vi "Send SYNC Pulse.vi"(8 "error in":errorcluster, 10 "Master?":bool=TRUE, 11 "FPGA Session":T1) -> (0 "error out":errorcluster, 3 "FPGA Session":T1)   [LabVIEW 2011, in "FlexRIO Host Library (User).lvlib"]
uses:
  FlexRIO Host Library (User).lvlib
  Session/FPGA Session Ref.ctl
  <vilib>/rvi/interface/nirviReadWriteControl/nirviReadWriteControl.xnode
  Zeiss Acquisition Demo/FPGA Bitfiles/FlexRIODigitizer_FPGABoard_Acquire_Rev2.lvbitx
  <vilib>/rvi/errors/niLvFpgaMergeErrorWithErrorCode.vi
  <vilib>/rvi/errors/niLvFpgaAdjustHostInterfaceError.vi
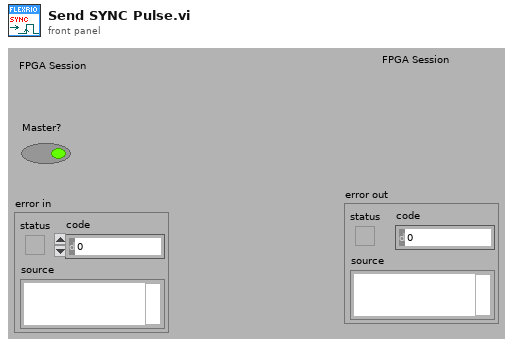
[diagram p1: front panel]
types:
  T1 = typedef "FlexRIO Host.lvlib/FPGA Session Ref.ctl" = refnum<k20>
  T2 = cluster{"Send SYNC Pulse":bool, "Send Software Start":bool}
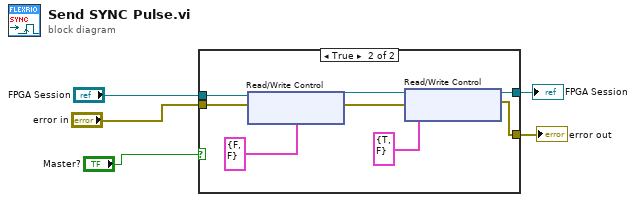
[diagram p0: block diagram]
diagram:
  n1 = case shown="True" "Master?" {
    tunnel: "FPGA Session" -> [w7 w15]
    tunnel: "error in" -> [w6 w14]
    tunnel: [w7 w11] -> w3
    tunnel: [w6 w10] -> w2
    frame False {
    }
    frame True {
      n2 = xnode "Read/Write Control"("FPGA VI Reference In"=w15, "error in"=w14, "Trigger Signals"=T2 {"Send SYNC Pulse"=FALSE, "Send Software Start"=FALSE}) -> ("FPGA VI Reference Out"=w13:T1, "error out"=w12:errorcluster)
      n3 = xnode "Read/Write Control"("FPGA VI Reference In"=w13, "error in"=w12, "Trigger Signals"=T2 {"Send SYNC Pulse"=TRUE, "Send Software Start"=FALSE}) -> ("FPGA VI Reference Out"=w11:T1, "error out"=w10:errorcluster)
    }
  }
  "error out" <- w2
  "FPGA Session" <- w3
